vi "Read Context.vi"(8 "error in (no error)":errorcluster, 11 "Network Stream in":refnum<class "Network Stream.lvclass">) -> (0 "error out":errorcluster, 2 "Context":string, 3 "Network Stream out":refnum<class "Network Stream.lvclass">)   [LabVIEW 2014, in "Network Stream.lvlib" / "Network Stream.lvclass"]
uses:
  Network Stream.lvclass
  Network Stream.lvclass/Network Stream.ctl
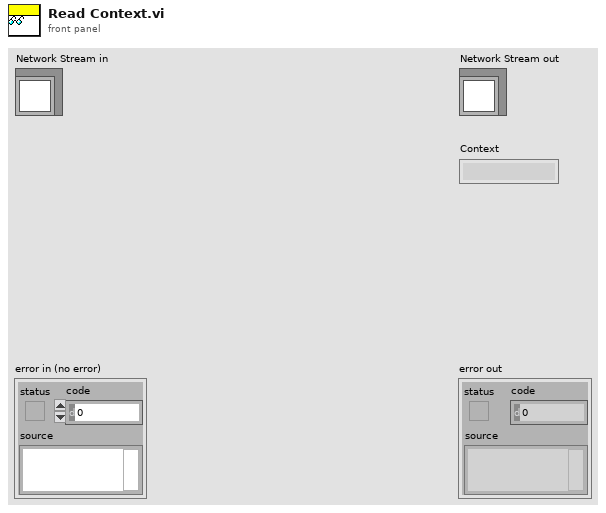
[diagram p1: front panel]
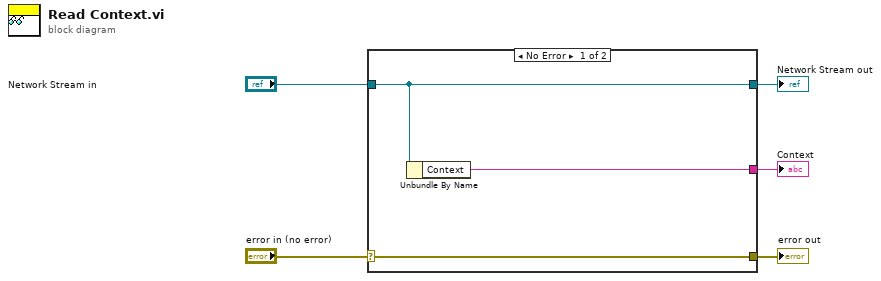
[diagram p0: block diagram]
diagram:
  n1 = case shown="No Error" "error in (no error)" {
    selector: "error in (no error)" -> [w8 w9]
    tunnel: [w8 w9] -> w4
    tunnel: [w7 w10] -> w2
    tunnel: "Network Stream in" -> [w7 w10]
    tunnel: [w6 _] -> w1
    frame No Error {
      n2 = Unbundle By Name(w7) -> ("Context"=w6:string)
    }
    frame Error {
    }
  }
  "error out" <- w4
  "Network Stream out" <- w2
  "Context" <- w1
